vi "Initialize Instrument.vi"(8 "error in (no error)":errorcluster, 10 "Reset":bool, 11 "VNA-ZNB in":refnum<class "VNA-ZNB.lvclass">) -> (0 "error out":errorcluster, 3 "VNA-ZNB out":refnum<class "VNA-ZNB.lvclass">)   [LabVIEW 2020, in "VNA-ZNB.lvclass"]
uses:
  VNA-ZNB.lvclass
  C:/Sandbox/Git_Sandbox/WiSpry Test Framework source code (LV20)/WiSpry Test Framework/Instruments/Instrument.lvclass
  C:/Sandbox/Git_Sandbox/WiSpry Test Framework source code (LV20)/WiSpry Test Framework/Instruments/Vector Network Analyzer/Vector Network Analyzer.lvclass
  <vilib>/Instr/_visa.llb/VISA Open Access Mode.ctl
  Instrument.lvclass/Instrument.ctl
  Vector Network Analyzer.lvclass/Vector Network Analyzer.ctl
  Instrument.lvclass
  Vector Network Analyzer.lvclass
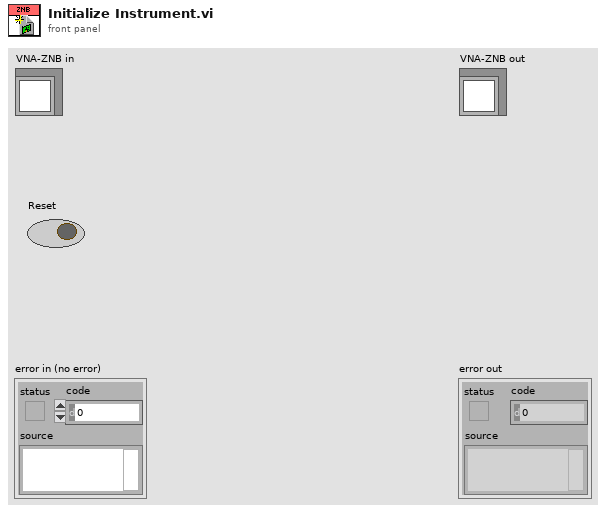
[diagram p1: front panel]
types:
  T1 = typedef "VISA Open Access Mode.ctl" = u32
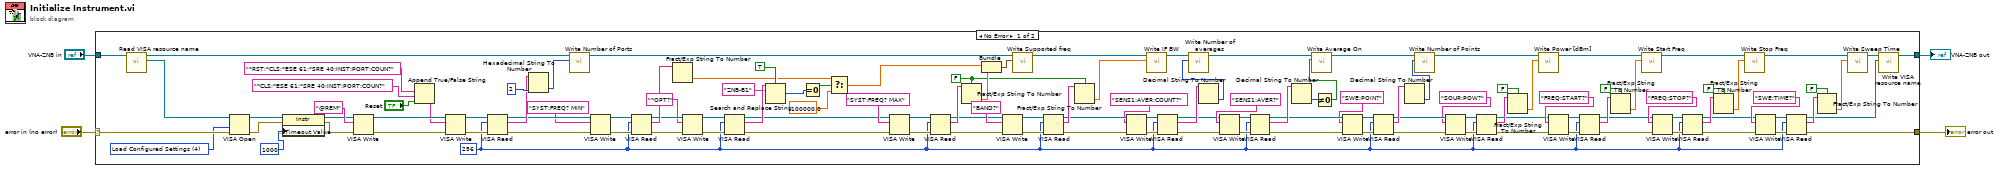
[diagram p0: block diagram]
diagram:
  n1 = case shown="No Error" "error in (no error)" {
    selector: "error in (no error)" -> [w128 w130]
    tunnel: "VNA-ZNB in" -> [w129 w131]
    tunnel: [w9 w130] -> w2
    tunnel: [w18 w131] -> w1
    frame No Error {
      w67 = FALSE ("use system decimal point (T)")
      w10 = u32 256 ("byte count")
      w126 = T1 4 items=["VISA Defaults"=0, "Exclusive Lock"=1, "Load Configured Settings"=4] ("Access Mode")
      n2 = call "Read VISA resource name.vi"("Instrument in"=w129) -> ("VISA resource name"=w127:refnum<visa-resource-name>, "Instrument out"=w122:refnum<class "VNA-ZNB.lvclass">)  [unwired: 9 in]
      n3 = VISA Open(access mode=w126, error in (no error)=w128, VISA resource name=w127) -> (VISA resource name=w124:refnum<visa-resource-name>, error out=w123:errorcluster)  [unwired: 2 in]
      n4 = property class="Instr"(reference=w124, error in=w123, "General Settings:Timeout Value"=u32 1000) -> (reference out=w118:refnum<visa-resource-name>, error out=w117:errorcluster)
      n5 = VISA Write(VISA resource name=w118, write buffer="@REM", error in (no error)=w117) -> (VISA resource name out=w115:refnum<visa-resource-name>, error out=w116:errorcluster)  [unwired: 1 out]
      n6 = Append True/False String(1:"Reset", 2:"*CLS;*ESE 61;*SRE 40;INST:PORT:COUN?" ("false string"), 3:"*RST;*CLS;*ESE 61;*SRE 40;INST:PORT:COUN?" ("Default Setup String")) -> (0:w112:string)  [unwired: 1 in]
      n7 = VISA Write(VISA resource name=w115, write buffer=w112, error in (no error)=w116) -> (VISA resource name out=w109:refnum<visa-resource-name>, error out=w110:errorcluster)  [unwired: 1 out]
      n8 = VISA Read(VISA resource name=w109, byte count=w10, error in (no error)=w110) -> (VISA resource name out=w107:refnum<visa-resource-name>, read buffer=w108:string, error out=w106:errorcluster)  [unwired: 1 out]
      n9 = Hexadecimal String To Number(string=w108, default (0uL)=2 ("default (0 U32)")) -> (number=w121:i32)  [unwired: 1 in, 1 out]
      n10 = call "Write Number of Ports.vi"("Number of Ports"=w121, "Vector Network Analyzer in"=w122) -> ("Vector Network Analyzer out"=w98:refnum<class "VNA-ZNB.lvclass">)  [unwired: 9 in]
      n11 = VISA Write(VISA resource name=w107, write buffer="SYST:FREQ? MIN", error in (no error)=w106) -> (VISA resource name out=w103:refnum<visa-resource-name>, error out=w104:errorcluster)  [unwired: 1 out]
      n12 = VISA Read(VISA resource name=w103, byte count=w10, error in (no error)=w104) -> (VISA resource name out=w88:refnum<visa-resource-name>, read buffer=w102:string, error out=w89:errorcluster)  [unwired: 1 out]
      n13 = Fract/Exp String To Number(string=w102) -> (number=w75:dbl)  [unwired: 3 in, 1 out]
      n14 = VISA Write(VISA resource name=w88, write buffer="*OPT?", error in (no error)=w89) -> (VISA resource name out=w85:refnum<visa-resource-name>, error out=w86:errorcluster)  [unwired: 1 out]
      n15 = VISA Read(VISA resource name=w85, byte count=w10, error in (no error)=w86) -> (VISA resource name out=w81:refnum<visa-resource-name>, read buffer=w83:string, error out=w82:errorcluster)  [unwired: 1 out]
      n16 = Search and Replace String(case sensitive?=TRUE ("ignore case? (F)"), input string=w83, search string="ZNB-B1") -> (number of replacements=w78:i32)  [unwired: 5 in, 3 out]
      n17 = Equal To 0?(x=w78) -> (x = 0?=w76:bool)
      n18 = Select(t=w75, s=w76, f=100000.0) -> (s? t:f=w77:dbl)
      n19 = VISA Write(VISA resource name=w81, write buffer="SYST:FREQ? MAX", error in (no error)=w82) -> (VISA resource name out=w100:refnum<visa-resource-name>, error out=w101:errorcluster)  [unwired: 1 out]
      n20 = VISA Read(VISA resource name=w100, byte count=w10, error in (no error)=w101) -> (VISA resource name out=w69:refnum<visa-resource-name>, read buffer=w99:string, error out=w70:errorcluster)  [unwired: 1 out]
      n21 = Fract/Exp String To Number(use system decimal point (T)=w67, string=w99) -> (number=w90:dbl)  [unwired: 2 in, 1 out]
      n22 = Bundle("f"=w77, w90) -> (w97:cluster{"f":dbl, dbl})  [unwired: 1 in]
      n23 = VISA Write(VISA resource name=w69, write buffer="BAND?", error in (no error)=w70) -> (VISA resource name out=w72:refnum<visa-resource-name>, error out=w71:errorcluster)  [unwired: 1 out]
      n24 = call "Write Supported freq.vi"("Supported freq"=w97, "Vector Network Analyzer in"=w98) -> ("Vector Network Analyzer out"=w19:refnum<class "VNA-ZNB.lvclass">)  [unwired: 9 in]
      n25 = VISA Read(VISA resource name=w72, byte count=w10, error in (no error)=w71) -> (VISA resource name out=w62:refnum<visa-resource-name>, read buffer=w68:string, error out=w63:errorcluster)  [unwired: 1 out]
      n26 = Fract/Exp String To Number(use system decimal point (T)=w67, string=w68) -> (number=w66:dbl)  [unwired: 2 in, 1 out]
      n27 = VISA Write(VISA resource name=w62, write buffer="SENS1:AVER:COUNT?", error in (no error)=w63) -> (VISA resource name out=w64:refnum<visa-resource-name>, error out=w65:errorcluster)  [unwired: 1 out]
      n28 = call "Write IF BW.vi"("IF BW"=w66, "Vector Network Analyzer in"=w19) -> ("Vector Network Analyzer out"=w96:refnum<class "VNA-ZNB.lvclass">)  [unwired: 9 in]
      n29 = VISA Read(VISA resource name=w64, byte count=w10, error in (no error)=w65) -> (VISA resource name out=w55:refnum<visa-resource-name>, read buffer=w60:string, error out=w54:errorcluster)  [unwired: 1 out]
      n30 = Decimal String To Number(string=w60) -> (number=w59:i32)  [unwired: 2 in, 1 out]
      n31 = call "Write Number of averages.vi"("Number of averages"=w59, "Vector Network Analyzer in"=w96) -> ("Vector Network Analyzer out"=w95:refnum<class "VNA-ZNB.lvclass">)  [unwired: 9 in]
      n32 = VISA Write(VISA resource name=w55, write buffer="SENS1:AVER?", error in (no error)=w54) -> (VISA resource name out=w57:refnum<visa-resource-name>, error out=w56:errorcluster)  [unwired: 1 out]
      n33 = VISA Read(VISA resource name=w57, byte count=w10, error in (no error)=w56) -> (VISA resource name out=w47:refnum<visa-resource-name>, read buffer=w53:string, error out=w48:errorcluster)  [unwired: 1 out]
      n34 = Decimal String To Number(string=w53) -> (number=w52:i32)  [unwired: 2 in, 1 out]
      n35 = Not Equal To 0?(x=w52) -> (x != 0?=w51:bool)
      n36 = call "Write Average On.vi"("Average On"=w51, "Vector Network Analyzer in"=w95) -> ("Vector Network Analyzer out"=w94:refnum<class "VNA-ZNB.lvclass">)  [unwired: 9 in]
      n37 = VISA Write(VISA resource name=w47, write buffer="SWE:POIN?", error in (no error)=w48) -> (VISA resource name out=w49:refnum<visa-resource-name>, error out=w50:errorcluster)  [unwired: 1 out]
      n38 = VISA Read(VISA resource name=w49, byte count=w10, error in (no error)=w50) -> (VISA resource name out=w41:refnum<visa-resource-name>, read buffer=w45:string, error out=w40:errorcluster)  [unwired: 1 out]
      n39 = Decimal String To Number(string=w45) -> (number=w44:i32)  [unwired: 2 in, 1 out]
      n40 = call "Write Number of Points.vi"("Number of Points"=w44, "Vector Network Analyzer in"=w94) -> ("Vector Network Analyzer out"=w93:refnum<class "VNA-ZNB.lvclass">)  [unwired: 9 in]
      n41 = VISA Write(VISA resource name=w41, write buffer="SOUR:POW?", error in (no error)=w40) -> (VISA resource name out=w43:refnum<visa-resource-name>, error out=w42:errorcluster)  [unwired: 1 out]
      n42 = VISA Read(VISA resource name=w43, byte count=w10, error in (no error)=w42) -> (VISA resource name out=w29:refnum<visa-resource-name>, read buffer=w38:string, error out=w30:errorcluster)  [unwired: 1 out]
      n43 = Fract/Exp String To Number(use system decimal point (T)=FALSE, string=w38) -> (number=w36:dbl)  [unwired: 2 in, 1 out]
      n44 = call "Write Power [dBm].vi"("Power [dBm]"=w36, "Vector Network Analyzer in"=w93) -> ("Vector Network Analyzer out"=w92:refnum<class "VNA-ZNB.lvclass">)  [unwired: 9 in]
      n45 = VISA Write(VISA resource name=w29, write buffer="FREQ:START?", error in (no error)=w30) -> (VISA resource name out=w31:refnum<visa-resource-name>, error out=w32:errorcluster)  [unwired: 1 out]
      n46 = VISA Read(VISA resource name=w31, byte count=w10, error in (no error)=w32) -> (VISA resource name out=w21:refnum<visa-resource-name>, read buffer=w34:string, error out=w22:errorcluster)  [unwired: 1 out]
      n47 = Fract/Exp String To Number(use system decimal point (T)=FALSE, string=w34) -> (number=w28:dbl)  [unwired: 2 in, 1 out]
      n48 = call "Write Start Freq.vi"("Start Freq"=w28, "Vector Network Analyzer in"=w92) -> ("Vector Network Analyzer out"=w91:refnum<class "VNA-ZNB.lvclass">)  [unwired: 9 in]
      n49 = VISA Write(VISA resource name=w21, write buffer="FREQ:STOP?", error in (no error)=w22) -> (VISA resource name out=w27:refnum<visa-resource-name>, error out=w26:errorcluster)  [unwired: 1 out]
      n50 = VISA Read(VISA resource name=w27, byte count=w10, error in (no error)=w26) -> (VISA resource name out=w11:refnum<visa-resource-name>, read buffer=w24:string, error out=w12:errorcluster)  [unwired: 1 out]
      n51 = Fract/Exp String To Number(use system decimal point (T)=FALSE, string=w24) -> (number=w20:dbl)  [unwired: 2 in, 1 out]
      n52 = call "Write Stop Freq.vi"("Stop Freq"=w20, "Vector Network Analyzer in"=w91) -> ("Vector Network Analyzer out"=w8:refnum<class "VNA-ZNB.lvclass">)  [unwired: 9 in]
      n53 = VISA Write(VISA resource name=w11, write buffer="SWE:TIME?", error in (no error)=w12) -> (VISA resource name out=w13:refnum<visa-resource-name>, error out=w14:errorcluster)  [unwired: 1 out]
      n54 = VISA Read(VISA resource name=w13, byte count=w10, error in (no error)=w14) -> (VISA resource name out=w5:refnum<visa-resource-name>, read buffer=w16:string, error out=w9:errorcluster)  [unwired: 1 out]
      n55 = Fract/Exp String To Number(use system decimal point (T)=FALSE, string=w16) -> (number=w6:dbl)  [unwired: 2 in, 1 out]
      n56 = call "Write Sweep Time.vi"("Sweep Time"=w6, "Vector Network Analyzer in"=w8) -> ("Vector Network Analyzer out"=w7:refnum<class "VNA-ZNB.lvclass">)  [unwired: 9 in]
      n57 = call "Write VISA resource name.vi"("VISA resource name"=w5, "Instrument in"=w7) -> ("Instrument out"=w18:refnum<class "VNA-ZNB.lvclass">)  [unwired: 9 in]
    }
    frame Error {
    }
  }
  "error out" <- w2
  "VNA-ZNB out" <- w1
